vi "LVCAM Create Nest.vi"(9 "Alias":string, 10 "Nest Actor":refnum<class "LVCAM.lvclass">, 11 "Self Actor in":refnum<class "Self Actor.lvclass">) -> (0 "error out":errorcluster, 3 "Self Actor out":refnum<class "Self Actor.lvclass">)   [LabVIEW 2021, in "LVCAM.lvlib" / "Self Actor.lvclass"]
uses:
  Self Actor.lvclass
  C:/PPLs/LabVIEW-Composed-Actor-Model-LVCAM/LabVIEW-Composed-Actor-Model-LVCAM/AAM/LVCAM/LVCAM/LVCAM.lvclass
  LVCAM/LVCAM.lvclass
  Self Actor.lvclass/Self Actor.ctl
  LVCAM/Msg Loop.vi
  Msg Q/Msg Q.lvclass
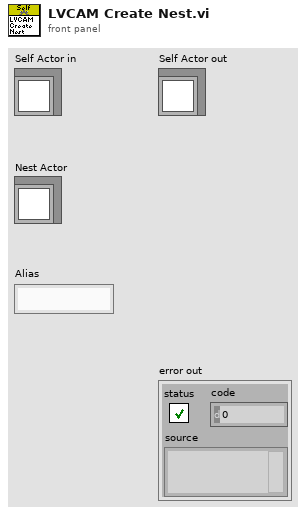
[diagram p1: front panel]
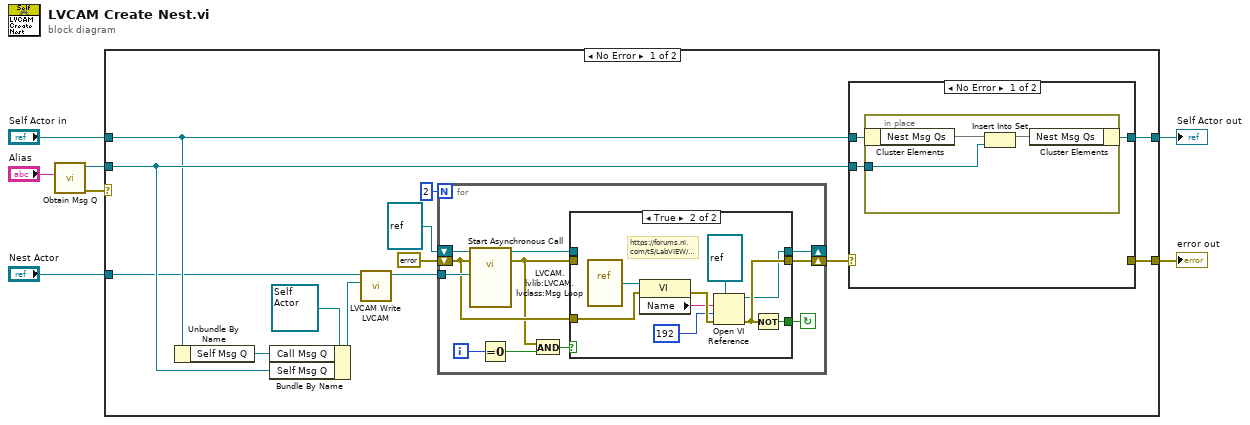
[diagram p0: block diagram]
diagram:
  n1 = call "Obtain Msg Q.vi"("Alias"="Alias") -> ("error out"=w1:errorcluster, "Msg Queue out"=w3:refnum<class "Msg Q.lvclass">)  [unwired: 9 in]
  n2 = case shown="No Error" w1 {
    selector: w1 -> [_ w52]
    tunnel: [w20 w51] -> w6
    tunnel: [w14 w52] -> w5
    tunnel: "Nest Actor" -> [w8 _]
    tunnel: w3 -> [w10 _]
    tunnel: "Self Actor in" -> [w9 w51]
    frame No Error {
      n3 = Unbundle By Name(w9) -> ("Self Msg Q"=w11:refnum<class "Msg Q.lvclass">)
      n4 = Bundle By Name(cluster=refnum<class "Self Actor.lvclass"> refnum ("Self Actor in"), "Call Msg Q"=w11, "Self Msg Q"=w10) -> (w12:refnum<class "Self Actor.lvclass">)
      n5 = call-dynamic "LVCAM Write LVCAM.vi"("LVCAM"=w12, "LVCAM Write LVCAM in"=w8) -> ("LVCAM Write LVCAM out"=w15:refnum<class "LVCAM.lvclass">)  [unwired: 9 in]
      n6 = for {
        N: 2 -> [_]
        tunnel: w15 -> [w39]
        shift-right: [w30] -> w19
        shift-left: errorcluster {"status"=FALSE, "code"=0, "source"=""} ("error out") -> [w33]
        shift-right: [w36] -> _
        shift-left: refnum<vi> refnum ("type specifier VI Refnum (for type only)") -> [w29]
        i -> [w38]
        stop <- w32 continue-if-true
        n7 = call-by-ref "Start Asynchronous Call"(reference=w29, error in=w33, "Actor in"=w39) -> (reference out=w35:refnum<vi>, error out=w31:errorcluster)  [unwired: 11 in]
        n8 = Equal To 0?(x=w38) -> (x = 0?=w37:bool)
        n9 = And(x=w31, y=w37) -> (x .and. y?=w34:bool)
        n10 = case shown="True" w34 {
          tunnel: [w40 w45] -> w36
          tunnel: w35 -> [w40 _]
          tunnel: w33 -> [_ w49]
          tunnel: w31 -> [w41 _]
          tunnel: [_ w50] -> w32
          tunnel: [w41 w46] -> w30
          frame False {
          }
          frame True {
            # "https://forums.ni.com/t5/LabVIEW/Static-VI-Reference/m-p/3334014#M978333"
            n11 = vi-ref "LVCAM.lvlib:LVCAM.lvclass:Msg Loop.vi"() -> (w42:refnum<vi>)
            n12 = property class="VI"(reference=w42, error in=w49) -> (error out=w48:errorcluster, "Name"=w47:string)  [unwired: 1 out]
            n13 = Open VI Reference(type specifier VI Refnum (for type only)=refnum<vi> refnum, vi path=w47, options=192 ("options: Multiple Clones,\n  Fire & Forget"), error in (no error)=w48) -> (vi reference=w45:refnum<vi>, error out=w46:errorcluster)  [unwired: 2 in]
            n14 = Not(x=w46) -> (.not. x?=w50:bool)
          }
        }
      }
      n15 = case shown="No Error" w19 {
        selector: w19 -> [_ w28]
        tunnel: w9 -> [w23 w27]
        tunnel: [w22 w27] -> w20
        tunnel: w10 -> [w21 _]
        tunnel: [_ w28] -> w14
        frame No Error {
          n16 = in-place {
            in-place-border: w21 -> [w24]
            n17 = in-place-cluster #1(w23) -> ("Nest Msg Qs"=w26:set{refnum<class "Msg Q.lvclass">})
            n18 = Insert Into Set(10:w24, 11:w26) -> (3:w25:set{refnum<class "Msg Q.lvclass">})  [unwired: 1 out]
            n19 = in-place-cluster #1("Nest Msg Qs"=w25) -> (w22:refnum<class "Self Actor.lvclass">)
          }
        }
        frame Error {
          # "#LVCAMError"
        }
      }
    }
    frame Error {
      # "#LVCAMError"
    }
  }
  "error out" <- w5
  "Self Actor out" <- w6
